vi "CalibrationDialog.vi"(4 "error in":errorcluster) -> (0 "error out":errorcluster, 3 "Yes?":bool)   [LabVIEW 2013]
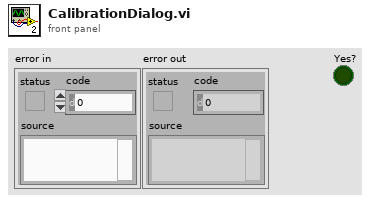
[diagram p1: front panel]
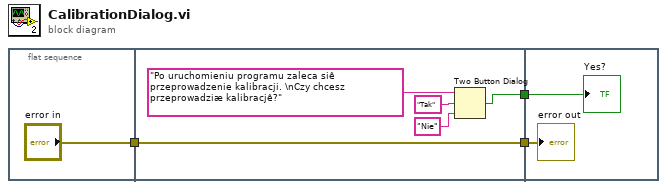
[diagram p0: block diagram]
diagram:
  n1 = flat-sequence {
    tunnel: ["error in"] -> w2
    tunnel: [w6] -> w3
    tunnel: w2 -> [w6]
    tunnel: [w5] -> w1
    tunnel: w3 -> [w11]
    tunnel: w1 -> [w10]
    frame #0 {
    }
    frame #1 {
      n2 = Two Button Dialog(message="Po uruchomieniu programu zaleca siê przeprowadzenie kalibracji. \nCzy chcesz przeprowadziæ kalibracjê?", 1:"Nie" ("F button name (\"Cancel\")"), 2:"Tak" ("T button name (\"OK\")")) -> (T button?=w5:bool)
    }
    frame #2 {
      "error out" <- w11
      "Yes?" <- w10
    }
  }
